vi "Image Process mk2.vi"(3 "error in":errorcluster, 5 "Image":T1) -> (0 "error out":errorcluster, 1 "Image Out":T1)   [LabVIEW 2011]
uses:
  <vilib>/vision/Image Controls.llb/IMAQ Image.ctl
  <vilib>/vision/NI_Vision_Development_Module.lvlib
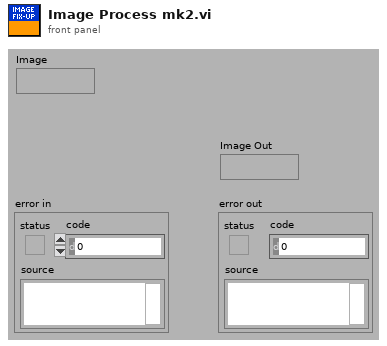
[diagram p1: front panel]
types:
  T1 = typedef "IMAQ Image.ctl" = refnum<image>
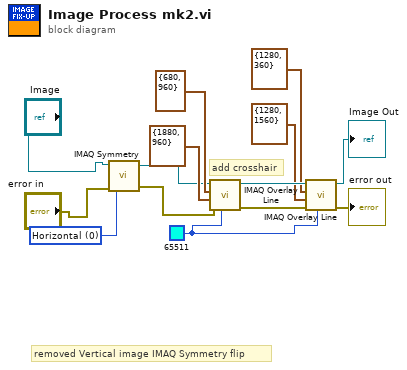
[diagram p0: block diagram]
diagram:
  w1 = u32 0 items=["Horizontal", "Vertical", "Central", "1st Diagonal", "2nd Diagonal"] ("Type of Symmetry")
  w14 = u32 65511 ("Color")
  # "removed Vertical image IMAQ Symmetry flip"
  # "add crosshair"
  n1 = call "IMAQ Symmetry"("error in (no error)"="error in", "Type of Symmetry"=w1, "Image Src"="Image") -> ("error out"=w2:errorcluster, "Image Dst Out"=w3:T1)  [unwired: 2 in]
  n2 = call "IMAQ Overlay Line"("Color"=w14, "error in (no error)"=w2, "End Point"=cluster{"X":i32, "Y":i32} {"X"=1880, "Y"=960}, "Start Point"=cluster{"X":i32, "Y":i32} {"X"=680, "Y"=960}, "Image"=w3) -> ("error out"=w8:errorcluster, "Image Out"=w13:T1)  [unwired: 1 in, 4 out]
  n3 = call "IMAQ Overlay Line"("Color"=w14, "error in (no error)"=w8, "End Point"=cluster{"X":i32, "Y":i32} {"X"=1280, "Y"=1560}, "Start Point"=cluster{"X":i32, "Y":i32} {"X"=1280, "Y"=360}, "Image"=w13) -> ("error out"=→"error out":errorcluster, "Image Out"=→"Image Out":T1)  [unwired: 1 in, 4 out]
